vi "Post-Install Custom Action.vi"(10 "Variant":variant) -> (0 "error out":errorcluster)   [LabVIEW 2014]
uses:
  <vilib>/Utility/sysdir.llb/System Directory Type.ctl
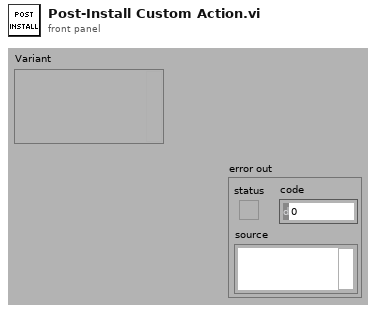
[diagram p1: front panel]
types:
  T1 = typedef "System Directory Type.ctl" = i32
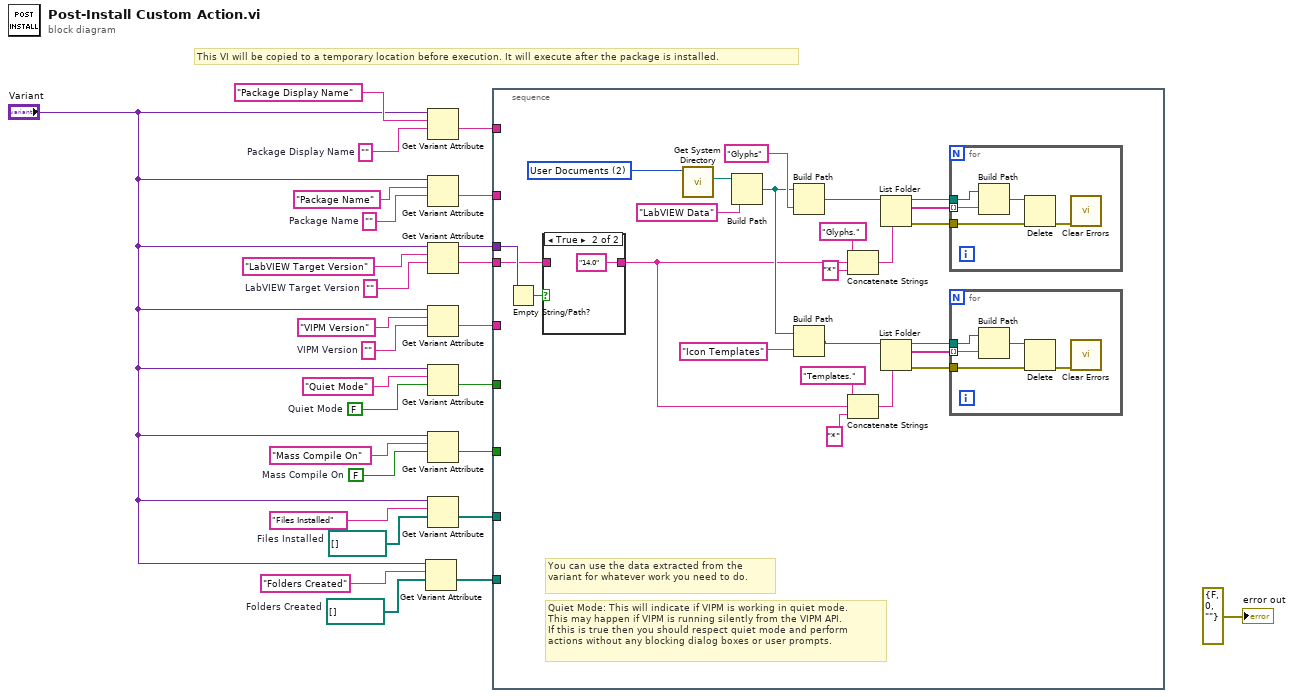
[diagram p0: block diagram]
diagram:
  w2 = path[] []  # Folders Created
  w3 = path[] []  # Files Installed
  w9 = FALSE  # Mass Compile On
  w10 = ""  # Package Display Name
  w17 = FALSE  # Quiet Mode
  w20 = ""  # VIPM Version
  w22 = ""  # LabVIEW Target Version
  w24 = ""  # Package Name
  # "This VI will be copied to a temporary location before execution. It will execute after the package is installed."
  n1 = Get Variant Attribute(Variant="Variant", name="Folders Created", default value (empty Variant)=w2) -> (value=w7:path[])  [unwired: 1 in, 3 out]
  n2 = Get Variant Attribute(Variant="Variant", name="Package Display Name", default value (empty Variant)=w10) -> (value=w16:string)  [unwired: 1 in, 3 out]
  n3 = Get Variant Attribute(Variant="Variant", name="Package Name", default value (empty Variant)=w24) -> (value=w15:string)  [unwired: 1 in, 3 out]
  n4 = Get Variant Attribute(Variant="Variant", name="LabVIEW Target Version", default value (empty Variant)=w22) -> (duplicate Variant=w1:variant, value=w14:string)  [unwired: 1 in, 2 out]
  n5 = Get Variant Attribute(Variant="Variant", name="VIPM Version", default value (empty Variant)=w20) -> (value=w13:string)  [unwired: 1 in, 3 out]
  n6 = Get Variant Attribute(Variant="Variant", name="Quiet Mode", default value (empty Variant)=w17) -> (value=w12:bool)  [unwired: 1 in, 3 out]
  n7 = Get Variant Attribute(Variant="Variant", name="Mass Compile On", default value (empty Variant)=w9) -> (value=w11:bool)  [unwired: 1 in, 3 out]
  n8 = Get Variant Attribute(Variant="Variant", name="Files Installed", default value (empty Variant)=w3) -> (value=w6:path[])  [unwired: 1 in, 3 out]
  n9 = stacked-sequence {
    tunnel: w16 -> [_]
    tunnel: w15 -> [_]
    tunnel: w14 -> [w28]
    tunnel: w13 -> [_]
    tunnel: w12 -> [_]
    tunnel: w11 -> [_]
    tunnel: w6 -> [_]
    tunnel: w7 -> [_]
    tunnel: w1 -> [w31]
    frame #0 {
      w51 = T1 2 items=["User Home"=0, "User Desktop"=1, "User Documents"=2, "User Application Data"=3, "User Preferences"=4, "User Temporary"=5, "Public Documents"=6, "Public Application Data"=7, "Public Preferences"=8, "Public Cache"=13, "System Core Libraries"=9, "System Installed Libraries"=10, "Application Files"=11, "Boot Volume Root"=12] ("system directory type")
      # "Quiet Mode: This will indicate if VIPM is working in quiet mode.\nThis may happen if VIPM is running silently from the VIPM API.\nIf this is true then you should respect quiet mode and perform\nactions without any blocking dialog boxes or user prompts."
      # "You can use the data extracted from the variant for whatever work you need to do."
      n10 = Empty String/Path?(string/path=w31) -> (empty?=w30:bool)
      n11 = case shown="True" w30 {
        tunnel: [w52 "14.0" ("LabVIEW Target Version")] -> w29
        tunnel: w28 -> [w52 _]
        frame False {
        }
        frame True {
        }
      }
      n12 = call <vilib>:"Get System Directory.vi"("system directory type"=w51) -> ("system directory"=w50:path)  [unwired: 10 in]
      n13 = Build Path(base path=w50, name or relative path="LabVIEW Data") -> (appended path=w47:path)
      n14 = Build Path(base path=w47, name or relative path="Glyphs") -> (appended path=w45:path)
      n15 = Build Path(base path=w47, name or relative path="Icon Templates") -> (appended path=w34:path)
      n16 = Concatenate Strings("Glyphs." ("pattern"), w29, "*" ("string")) -> (w43:string)
      n17 = Concatenate Strings("Templates." ("pattern"), w29, "*" ("string")) -> (w36:string)
      n18 = List Folder(path=w45, pattern=w43) -> (path out=w41:path, filenames=w42:string[], error out=w40:errorcluster)  [unwired: 2 in, 1 out]
      n19 = List Folder(path=w34, pattern=w36) -> (path out=w38:path, filenames=w37:string[], error out=w39:errorcluster)  [unwired: 2 in, 1 out]
      n20 = for {
        tunnel: w42 -> [w63] mode=indexing
        tunnel: w41 -> [w62]
        tunnel: w40 -> [w60]
        n21 = Build Path(base path=w62, name or relative path=w63) -> (appended path=w61:path)
        n22 = Delete(path (use dialog)=w61, error in=w60) -> (error out=w59:errorcluster)  [unwired: 3 in, 2 out]
        n23 = call <vilib>:"Clear Errors.vi"("error in (no error)"=w59) -> ()  [unwired: 6 in, 1 out]
      }
      n24 = for {
        tunnel: w37 -> [w58] mode=indexing
        tunnel: w38 -> [w57]
        tunnel: w39 -> [w55]
        n25 = Build Path(base path=w57, name or relative path=w58) -> (appended path=w56:path)
        n26 = Delete(path (use dialog)=w56, error in=w55) -> (error out=w54:errorcluster)  [unwired: 3 in, 2 out]
        n27 = call <vilib>:"Clear Errors.vi"("error in (no error)"=w54) -> ()  [unwired: 6 in, 1 out]
      }
    }
  }
  "error out" <- errorcluster {"status"=FALSE, "code"=0, "source"=""} ("error out")
